vi "BRig_dataRT_stats__BTPR_avg_R.vi"() -> (2 "output_BTPR_avg_R__x100":i32)   [LabVIEW 2014]
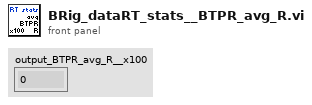
[diagram p1: front panel]
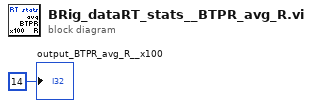
[diagram p0: block diagram]
diagram:
  "output_BTPR_avg_R__x100" <- 14 ("output_iBlock")
